vi "DMM_Scan DER Close.vi"(0 "Scan Resources Handles In":T1={"DMM Handle"="", "DAQmx Task Out"="", "Relays Status Array"=[], "N Shift Shunt"=1, "Close all Shunts?"=TRUE, "Relays Debounce Time (ms)"=5} caption="Scan Resource Handles In", 11 "error in":errorcluster) -> (15 "error out":errorcluster)   [LabVIEW 2021, in "DMM_Scan DAQ Ext RLY.lvlib"]
doc: "Opens all relays and closes the DAQmx and NI-DMM Scan session specifed in Scan Resource DMM Handles In, and releases all resources."
uses:
  DMM_Scan DAQ Ext RLY.lvlib
  Typedefs/Scan Resource Handles In.ctl
  DMM Mixed Measurements/DMM_Mixed Measurement.lvlib
  Static Digital State Generation/DAQ_Static Digital State Generation.lvlib
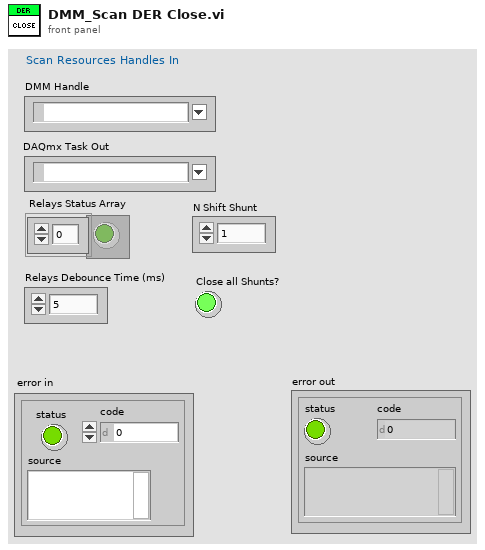
[diagram p1: front panel]
types:
  T1 = typedef "DMM_Scan DAQ Ext RLY.lvlib/Scan Resource Handles In.ctl" = cluster{"DMM Handle":refnum<k15>, "DAQmx Task Out":refnum<k21>, "Relays Status Array":bool[], "N Shift Shunt":u32, "Close all Shunts?":bool, "Relays Debounce Time (ms)":u32}
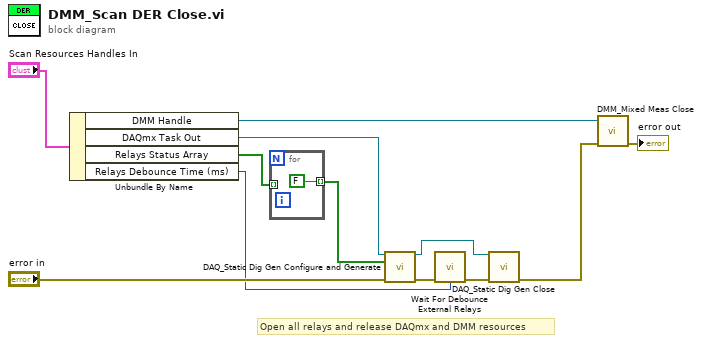
[diagram p0: block diagram]
diagram:
  # "Open all relays and release DAQmx and DMM resources"
  n1 = Unbundle By Name("Scan Resources Handles In") -> ("DMM Handle"=w11:refnum<k15>, "DAQmx Task Out"=w6:refnum<k21>, "Relays Status Array"=w8:bool[], "Relays Debounce Time (ms)"=w2:u32)
  n2 = for {
    tunnel: [FALSE] -> w1 mode=indexing
    tunnel: w8 -> [_] mode=indexing
  }
  n3 = call "DAQ_Static Dig Gen Configure and Generate.vi"("DAQmx Task In"=w6, "Data to Write"=w1, "error in"="error in") -> ("DAQmx Task Out"=w5:refnum<k21>, "error out"=w7:errorcluster)  [unwired: 10 in, 1 out]
  n4 = call "Wait For Debounce External Relays.vi"("error in"=w7, "Wait (ms)"=w2) -> ("error out"=w4:errorcluster)  [unwired: 13 in]
  n5 = call "DAQ_Static Dig Gen Close.vi"("DAQmx Task In"=w5, "error in"=w4) -> ("error out"=w10:errorcluster)  [unwired: 13 in]
  n6 = call "DMM_Mixed Meas Close.vi"("DMM Handle In"=w11, "error in"=w10) -> ("error out"=→"error out":errorcluster)  [unwired: 13 in]
